vi "BL132CameraPortal3.vi"() -> ()   [LabVIEW 2019]
panel:
  in  "APX_BEAM":bool
  in  "APX_PREP_TOP":bool=TRUE
  in  "APX_PREP_SIDE":bool=TRUE
  in  "APX_HPC_BOTTOM":bool=TRUE
  in  "APX_HPC_SIDE":bool=TRUE
  out "x = y?":bool
  in  "stop":bool
  in  "Tab Control":enum32{"PREP", "MAIN", "BEAM"}(tab)
  out "APX PREP TOP":T1(plugin-control)
  out "APX Sample Top View in PREP":T1(plugin-control)
  out "APX Sample Side View in PREP":T1(plugin-control)
  out "APX PREP SIDE":T1(plugin-control)
  out "APX HPC BOTTOM OV":T1(plugin-control)
  out "APX HPC BOTTOM APERTURE":T1(plugin-control)
  out "APX HPC SIDE EDGE":T1(plugin-control)
  out "APX HPC SIDE CONE":T1(plugin-control)
  out "APX HPC SIDE OV":T1(plugin-control)
  out "APX_BEAM":T1(plugin-control)
  out "BL132 BEAM":T1(plugin-control)
  out "error out":errorcluster
  in  "error in":errorcluster
  # "26u/pixel"
  # "0.5mm"
  # "12mm"
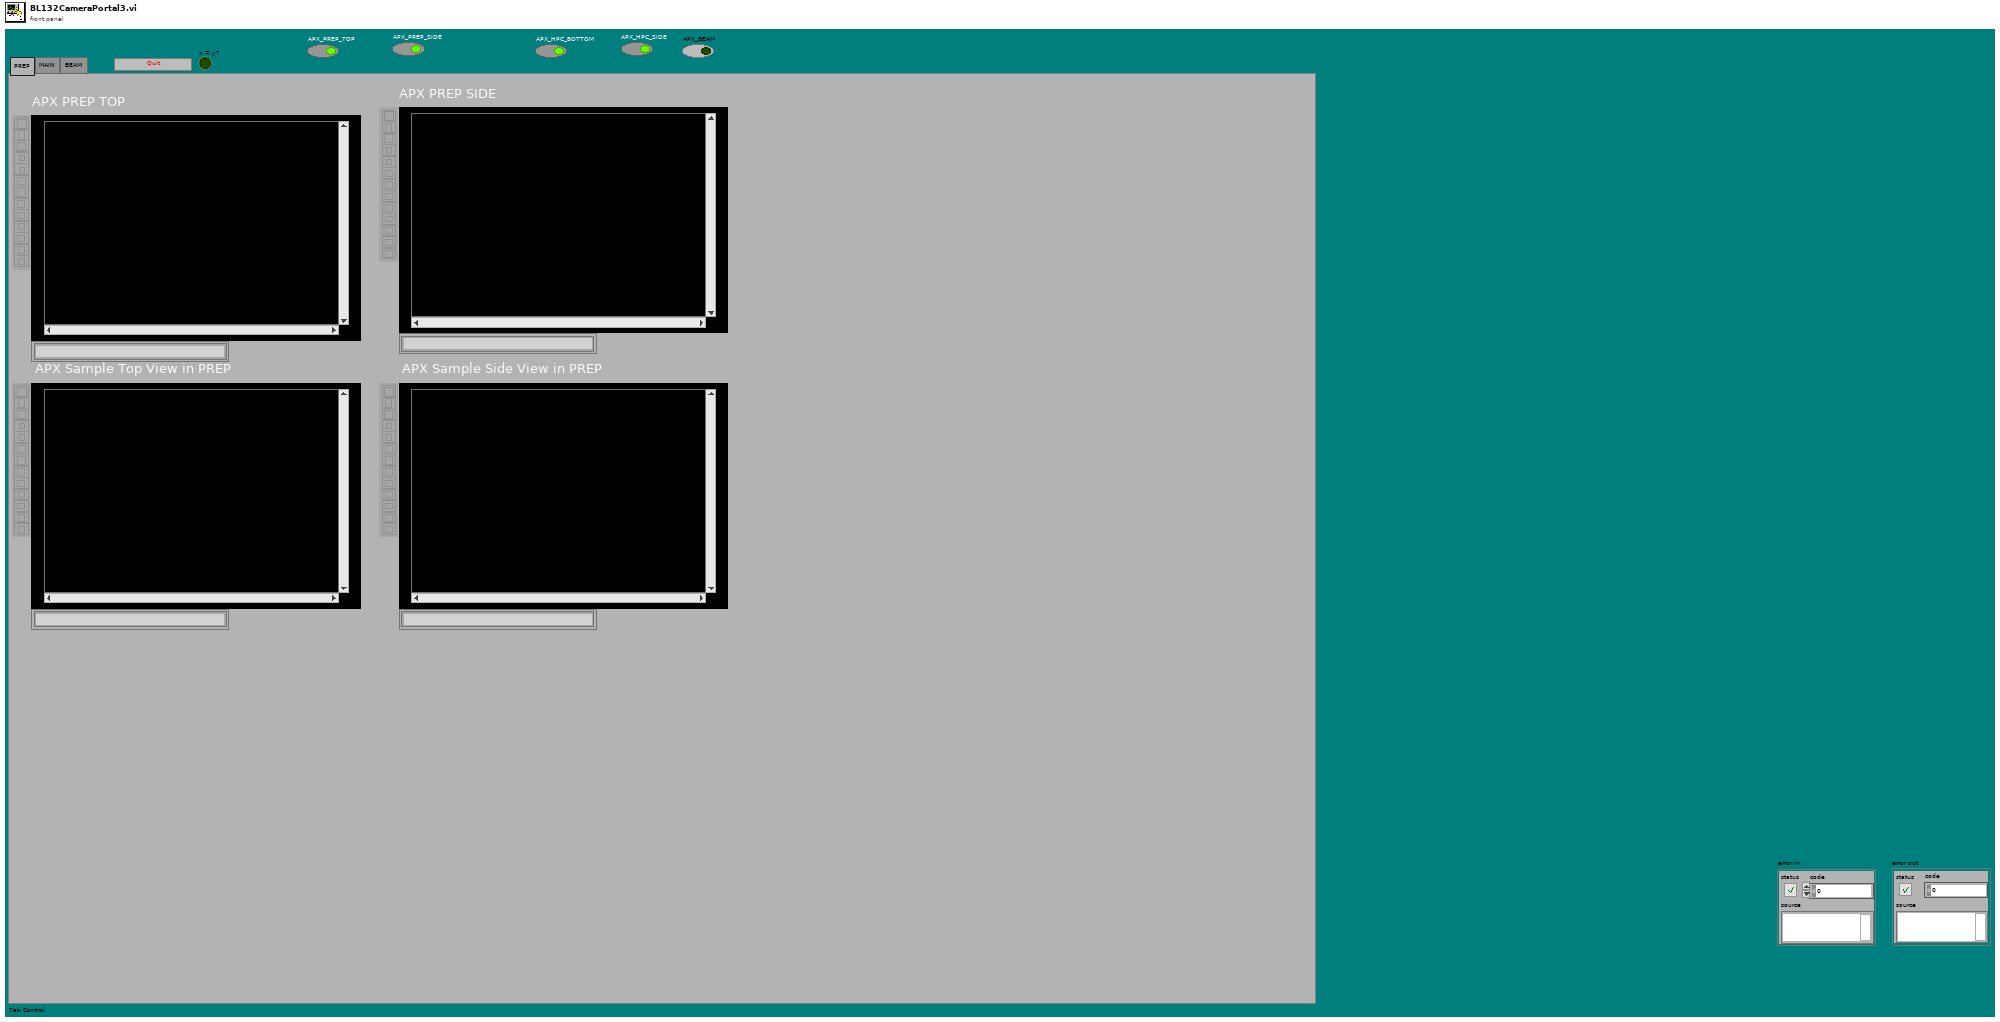
[diagram p1: front panel]
types:
  T1 = typedef "IMAQ Image.ctl" = refnum<image>
  T2 = cluster{"Pattern":i32, "Algorithm":i32, "Red Gain":dbl, "Green Gain":dbl, "Blue Gain":dbl}
  T3 = typedef "Image Type" = u32
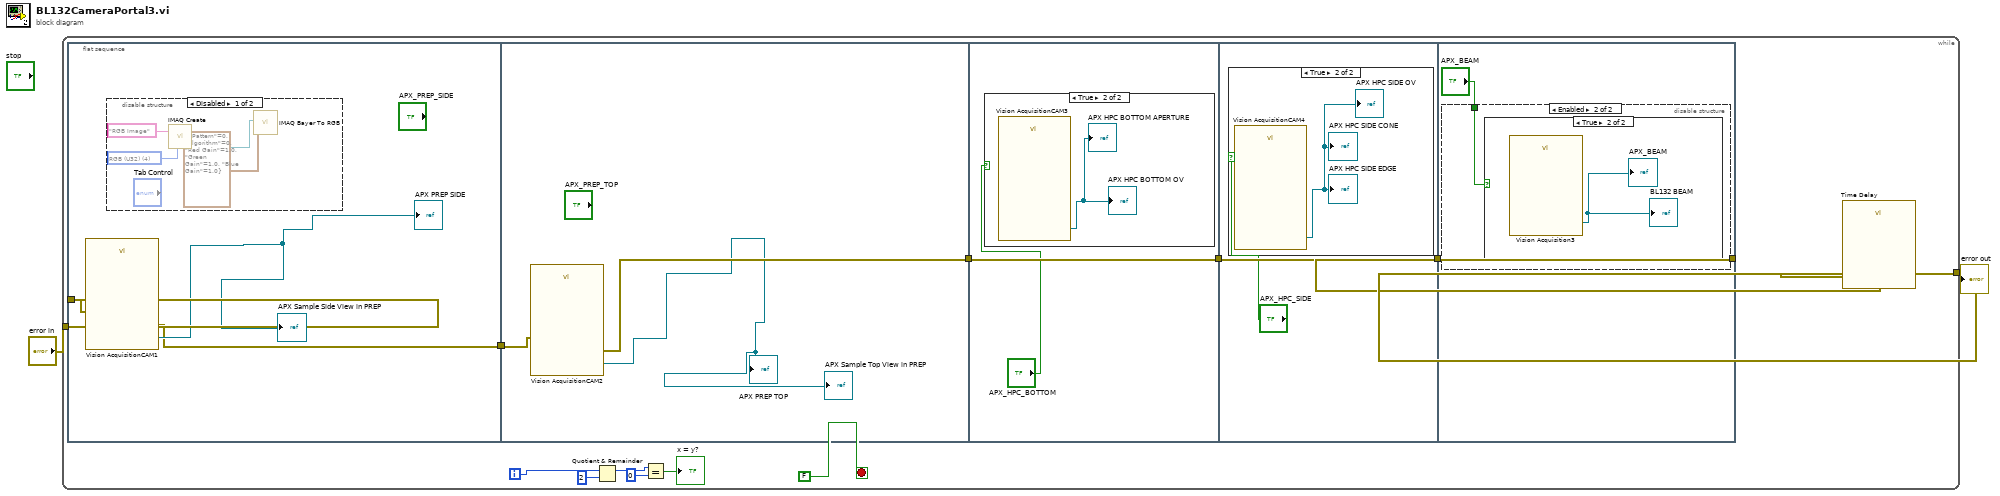
[diagram p0: block diagram]
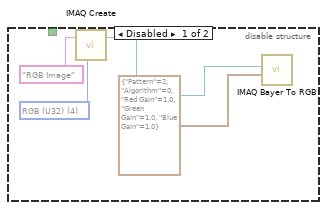
[diagram p5: hidden frame]
diagram:
  n1 = while {
    tunnel: [w9] -> w2
    tunnel: "error in" -> [w7]
    i -> [w14]
    stop <- FALSE stop-if-true
    n2 = flat-sequence {
      tunnel: [w17] -> w8
      tunnel: w7 -> [w16]
      tunnel: w8 -> [w25]
      tunnel: [w24] -> w6
      tunnel: w6 -> [w27]
      tunnel: [w27] -> w4
      tunnel: w4 -> [w30]
      tunnel: [w30] -> w3
      tunnel: [w33] -> w5
      tunnel: w3 -> [w33]
      frame #0 {
        n3 = call "Vision AcquisitionCAM1"("error in"=w16) -> ("Image Out"=→"APX Sample Side View in PREP" →"APX PREP SIDE":T1, "error out"=w17:errorcluster)  [unwired: 25 in]
        n4 = disable-structure shown="Disabled" {
          frame Disabled {
            w20 = T3 4 items=["Grayscale (U8)", "Grayscale (I16)", "Grayscale (SGL)", "Complex (CSG)", "RGB (U32)", "HSL (U32)", "RGB (U64)", "Grayscale (U16)"] ("Image Type")
            n5 = call "IMAQ Create"("Image Name"="RGB Image", "Image Type"=w20) -> ("New Image"=w19:T1)  [unwired: 2 in, 2 out]
            n6 = call "IMAQ Bayer To RGB"("Bayer Parameters"=T2 {"Pattern"=0, "Algorithm"=0, "Red Gain"=1.0, "Green Gain"=1.0, "Blue Gain"=1.0}, "Image Dst"=w19) -> ()  [unwired: 8 in, 2 out]
          }
          frame Enabled {
          }
        }
      }
      frame #1 {
        n7 = call "Vision AcquisitionCAM2"("error in"=w25) -> ("Image Out"=→"APX Sample Top View in PREP" →"APX PREP TOP":T1, "error out"=w24:errorcluster)  [unwired: 25 in]
      }
      frame #2 {
        n8 = case shown="True" "APX_HPC_BOTTOM" {
          frame False {
          }
          frame True {
            n9 = call "Vision AcquisitionCAM3"() -> ("Image Out"=→"APX HPC BOTTOM APERTURE" →"APX HPC BOTTOM OV":T1)  [unwired: 25 in, 2 out]
          }
        }
      }
      frame #3 {
        n10 = case shown="True" "APX_HPC_SIDE" {
          frame False {
          }
          frame True {
            n11 = call "Vision AcquisitionCAM4"() -> ("Image Out"=→"APX HPC SIDE OV" →"APX HPC SIDE CONE" →"APX HPC SIDE EDGE":T1)  [unwired: 25 in, 2 out]
          }
        }
      }
      frame #4 {
        n12 = disable-structure shown="Enabled" {
          disable-tunnel: "APX_BEAM" -> [_ w40]
          frame Disabled {
            w37 = T3 4 items=["Grayscale (U8)", "Grayscale (I16)", "Grayscale (SGL)", "Complex (CSG)", "RGB (U32)", "HSL (U32)", "RGB (U64)", "Grayscale (U16)"] ("Image Type")
            n13 = call "IMAQ Create"("Image Name"="RGB Image", "Image Type"=w37) -> ("New Image"=w36:T1)  [unwired: 2 in, 2 out]
            n14 = call "IMAQ Bayer To RGB"("Bayer Parameters"=T2 {"Pattern"=2, "Algorithm"=0, "Red Gain"=1.0, "Green Gain"=1.0, "Blue Gain"=1.0}, "Image Dst"=w36) -> ("Image Dst Out"=w34:T1, "Image Src"=w35:T1)  [unwired: 7 in, 1 out]
          }
          frame Enabled {
            n15 = case shown="True" w40 {
              frame False {
              }
              frame True {
                n16 = call "Vision Acquisition3"() -> ("Image Out"=→"APX_BEAM" →"BL132 BEAM":T1)  [unwired: 26 in, 1 out]
              }
            }
          }
        }
      }
    }
    n17 = Quotient & Remainder(x=w14, y=2) -> (x-y*floor(x/y)=w12:i32)  [unwired: 1 out]
    n18 = Equal?(x=w12, y=0) -> (x = y?=→"x = y?":bool)
    n19 = call "Time Delay"("error in (no error)"=w5) -> ("error out"=w9:errorcluster)  [unwired: 10 in]
  }
  "error out" <- w2
